vi "Wait Until Analog Count.vi"(0 "Device ID":T4(ring), 2 "Wait Until":T2(ring), 5 "Module":T1(ring), 7 "Analog_Input":T3(ring), 9 "Final Count":u32=1, 11 "error in":errorcluster, 12 "Level":dbl, 13 "Time Out (10)":dbl=10.0) -> (4 "Device ID Out":T4(ring), 15 "error out":errorcluster)   [LabVIEW 2010]
doc: "This VI waits until a specified number of user-defined analog edges are read."
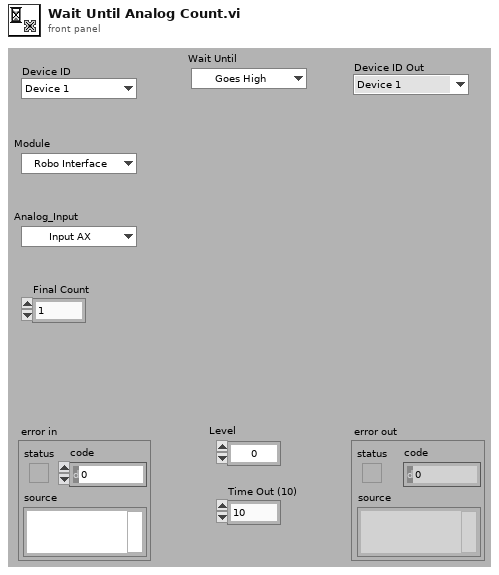
[diagram p1: front panel]
types:
  T1 = enum8{"Robo Interface", "Extension 1", "Extension 2", "Extension 3"}
  T2 = enum8{"Goes High", "Goes Low", "Goes High or Low"}
  T3 = enum8{"Input AX", "Input AY", "Input A1", "Input A2", "Input AZ", "Input AV", "Input D1", "Input D2", "Input AXR", "Input AYR"}
  T4 = enum16{"Device 1", "Device 2", "Device 3", "Device 4", "Device 5", "Device 6", "Device 7", "Device 8"}
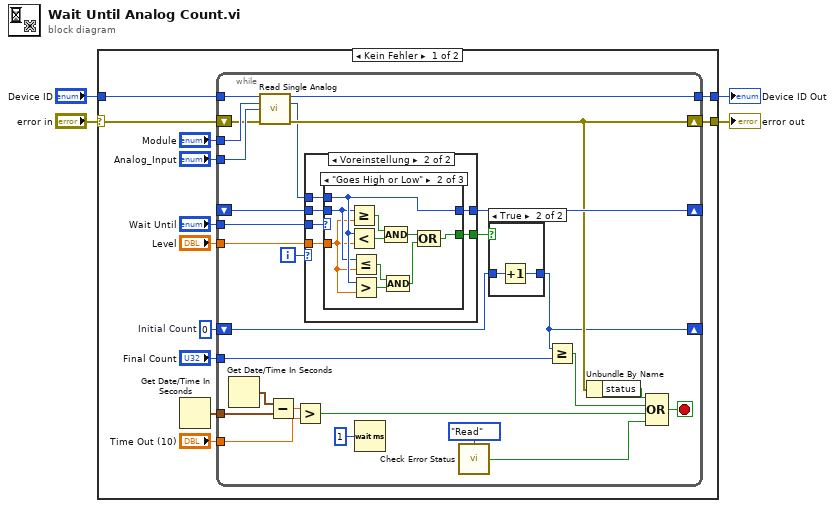
[diagram p0: block diagram]
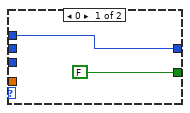
[diagram p3: hidden frame]
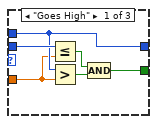
[diagram p4: hidden frame]
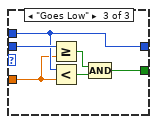
[diagram p5: hidden frame]
diagram:
  n1 = case shown="Kein Fehler" "error in" {
    selector: "error in" -> [w9 w78]
    tunnel: [w8 w78] -> w3
    tunnel: "Device ID" -> [w11 w77]
    tunnel: [w10 w77] -> w1
    frame No Error {
      w7 = u32 0  # Initial Count
      n2 = Get Date/Time In Seconds() -> (seconds since 1Jan1904=w15:timestamp)
      n3 = while {
        tunnel: "Wait Until" -> [w43]
        shift-right: [w37] -> _
        shift-left: _ -> [w36]
        tunnel: w15 -> [w41]
        tunnel: "Time Out (10)" -> [w39]
        tunnel: w11 -> [w32]
        tunnel: "Module" -> [w31]
        tunnel: "Analog_Input" -> [w30]
        tunnel: [w29] -> w10
        shift-right: [w27] -> w8
        shift-left: w9 -> [w28]
        shift-right: [w21] -> _
        shift-left: w7 -> [w24]
        tunnel: "Final Count" -> [w22]
        tunnel: "Level" -> [w20]
        i -> [w38]
        stop <- w34 stop-if-true
        n4 = Get Date/Time In Seconds() -> (seconds since 1Jan1904=w42:timestamp)
        n5 = call "Read Single Analog.vi"("Device ID"=w32, "Module"=w31, "Analog_Input"=w30, "error in"=w28) -> ("Device ID Out"=w29:T4, "Value"=w19:u16, "error out"=w27:errorcluster)  [unwired: 9 out]
        n6 = Subtract(x=w42, y=w41) -> (x-y=w40:dbl)
        n7 = Greater?(x=w40, y=w39) -> (0:w35:bool)
        n8 = case shown="Voreinstellung" w38 {
          tunnel: w43 -> [_ w54]
          tunnel: [w47 w52] -> w37
          tunnel: w36 -> [_ w53]
          tunnel: [FALSE w51] -> w25
          tunnel: w19 -> [w47 w50]
          tunnel: w20 -> [_ w49]
          frame 0 {
          }
          frame Default {
            n9 = case shown="\"Goes High or Low\"" w54 {
              tunnel: w53 -> [w60 w65 w74]
              tunnel: [w56 w66 w72] -> w52
              tunnel: [w57 w62 w73] -> w51
              tunnel: w50 -> [w56 w66 w72]
              tunnel: w49 -> [w55 w61 w71]
              frame "Goes High" {
                n10 = Less Or Equal?(x=w60, y=w55) -> (x <= y?=w59:bool)
                n11 = Greater?(x=w56, y=w55) -> (0:w58:bool)
                n12 = Compound Arithmetic op=AND(w59, w58) -> (w57:bool)
              }
              frame "Goes High or Low" {
                n13 = Greater Or Equal?(x=w65, y=w61) -> (x >= y?=w70:bool)
                n14 = Less?(x=w66, y=w61) -> (x < y?=w69:bool)
                n15 = Less Or Equal?(x=w65, y=w61) -> (x <= y?=w68:bool)
                n16 = Greater?(x=w66, y=w61) -> (0:w67:bool)
                n17 = Compound Arithmetic op=AND(w70, w69) -> (w64:bool)
                n18 = Compound Arithmetic op=AND(w68, w67) -> (w63:bool)
                n19 = Compound Arithmetic op=OR(w64, w63) -> (w62:bool)
              }
              frame "Goes Low" {
                n20 = Greater Or Equal?(x=w74, y=w71) -> (x >= y?=w76:bool)
                n21 = Less?(x=w72, y=w71) -> (x < y?=w75:bool)
                n22 = Compound Arithmetic op=AND(w76, w75) -> (w73:bool)
              }
            }
          }
        }
        n23 = Wait (ms)(milliseconds to wait=u32 1) -> ()  [unwired: 1 out]
        n24 = call "Check Error Status.vi"("Action (Write)"=enum16{"Write", "Read"}."Read") -> ("Error?"=w18:bool)  [unwired: 2 in, 12 out]
        n25 = case shown="TRUE" w25 {
          tunnel: [w44 w45] -> w21
          tunnel: w24 -> [w44 w46]
          frame False {
          }
          frame True {
            n26 = Increment(x=w46) -> (x+1=w45:u32)
          }
        }
        n27 = Greater Or Equal?(x=w21, y=w22) -> (x >= y?=w23:bool)
        n28 = Unbundle By Name(w27) -> ("status"=w26:bool)
        n29 = Compound Arithmetic op=OR(w26, w23, w35, w18) -> (w34:bool)
      }
    }
    frame Error {
    }
  }
  "error out" <- w3
  "Device ID Out" <- w1
